vi "Write to Display.vi"(8 "error in (no error)":errorcluster, 11 "Hardware Screen Interface in":refnum<class "Hardware Screen Interface.lvclass">) -> (0 "error out":errorcluster, 3 "Hardware Screen Interface out":refnum<class "Hardware Screen Interface.lvclass">)   [LabVIEW 2017, in "Hardware Screen Interface.lvlib" / "Hardware Screen Interface.lvclass"]
uses:
  Hardware Screen Interface.lvclass
  Hardware Screen Interface.lvclass/Hardware Screen Interface.ctl
  <vilib>/Utility/error.llb/Error Cluster From Error Code.vi
  <vilib>/rvi/errors/niLvFpgaAdjustHostInterfaceError.vi
  <vilib>/rvi/interface/nirviReadWriteControl/nirviReadWriteControl.xnode
  NiFpgaLv.dll
  <vilib>/rvi/interface/Simulation/niFpgaSimulationCallBeginRW.vi
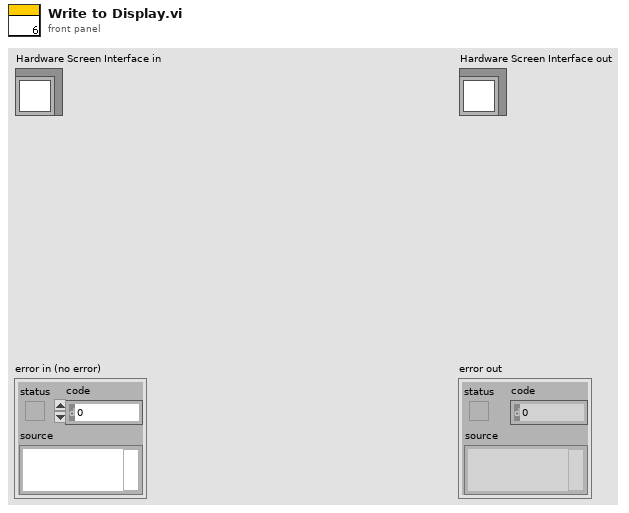
[diagram p1: front panel]
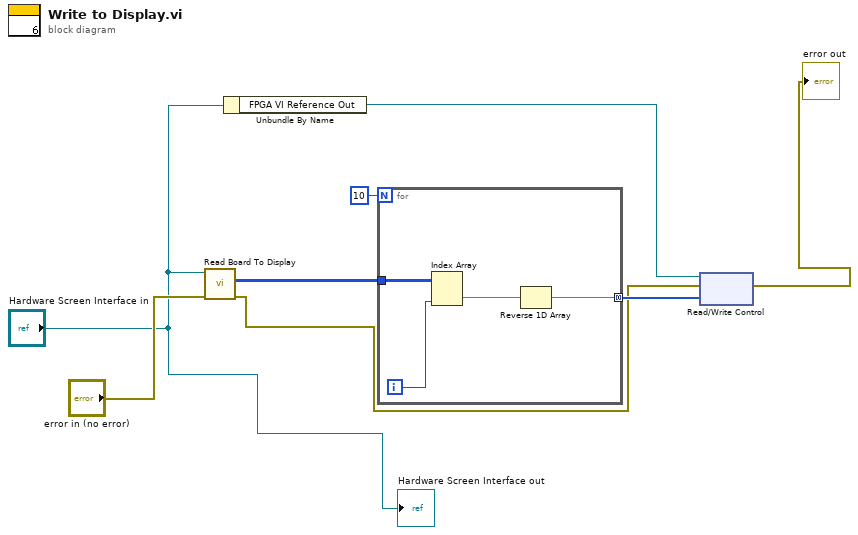
[diagram p0: block diagram]
diagram:
  n1 = call-dynamic "Read Board To Display.vi"("error in (no error)"="error in (no error)", "Screen Interface in"="Hardware Screen Interface in") -> ("error out"=w2:errorcluster, "Board To Display"=w7:u32[][])  [unwired: 7 in, 1 out]
  n2 = Unbundle By Name("Hardware Screen Interface in") -> ("FPGA VI Reference Out"=w4:refnum<k20>)
  n3 = for {
    N: 10 -> [_]
    tunnel: w7 -> [w12]
    tunnel: [w9] -> w3 mode=concatenating
    i -> [w10]
    n4 = Index Array(array=w12, index (col)=w10) -> (element=w11:u32[])  [unwired: 1 in]
    n5 = Reverse 1D Array(array=w11) -> (reversed array=w9:u32[])
  }
  n6 = xnode "Read/Write Control"("FPGA VI Reference In"=w4, "error in"=w2, "u"=w3) -> ("error out"=→"error out":errorcluster)  [unwired: 1 out]
  "Hardware Screen Interface out" <- "Hardware Screen Interface in"
